vi "Check BOM against Inventory.vi"() -> ()   [LabVIEW 2013]
panel:
  out "Report":string
  in  "Check":bool
  in  "BOM":path
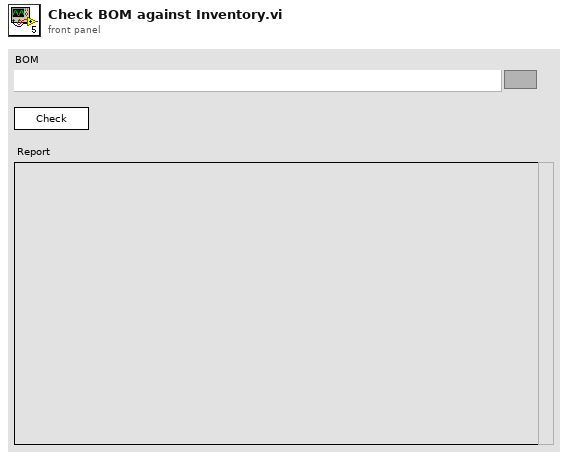
[diagram p1: front panel]
types:
  T1 = typedef "Display Component Line.ctl" = cluster{"Part Number":string, "Code (Value)":string, "Component Type":T2, "Component Subtype":T3, "Quantity":u32, "Add":T4, "Subtract":T5}
  T2 = typedef "Components.ctl" = enum16{"Resistor", "Capacitor", "Diode", "Voltage Regulator", "Transistors", "ICs", "Misc"}
  T3 = typedef "Component Sub Type.ctl" = enum16{"N/A", "Carbon", "Variable - Trimmer", "Variable - Pot", "Ceramic", "Electrolitic", "Zenner", "TO-92", "TO-220", "NPN", "PNP", "CMOS", "Processor"}
  T4 = typedef "Add Button.ctl" = bool
  T5 = typedef "Subtract Button.ctl" = bool
  T6 = typedef "BOM Item.ctl" = cluster{"Quantity":i32, "Component Type":string, "Component Value":string, "Component Type Estimate":T2, "Component Subtype Estimate":T3}
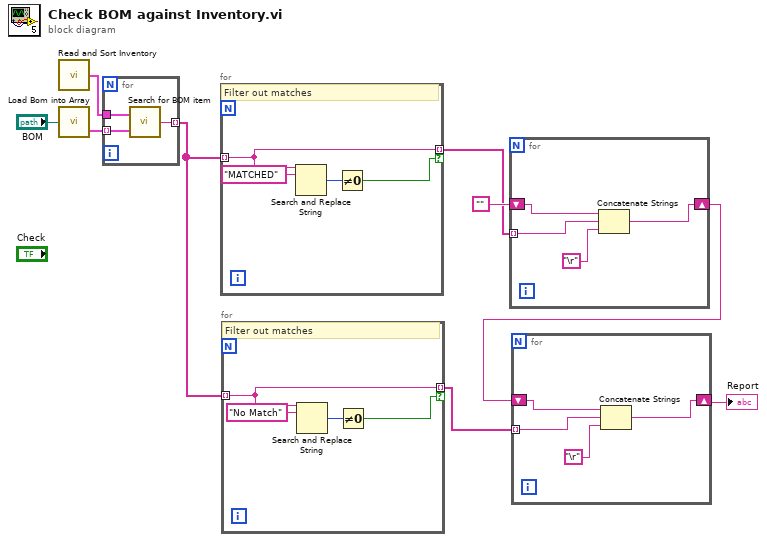
[diagram p0: block diagram]
diagram:
  n1 = call "Read and Sort Inventory.vi"() -> ("Array"=w7:T1[])  [unwired: 1 in]
  n2 = call "Load Bom into Array.vi"("BOM"="BOM") -> ("Cluster Bom"=w8:T6[])  [unwired: 1 out]
  n3 = for {
    tunnel: w8 -> [w12] mode=indexing
    tunnel: w7 -> [w11]
    tunnel: [w10] -> w6 mode=indexing
    n4 = call "Search for BOM item.vi"("BOM Item"=w12, "Inventory"=w11) -> ("Line Item Report"=w10:string)
  }
  n5 = for {
    tunnel: w6 -> [w14] mode=indexing
    tunnel: [w14] -> w4 mode=indexing if=w13
    # "Filter out matches"
    n6 = Search and Replace String(input string=w14, search string="MATCHED") -> (number of replacements=w15:i32)  [unwired: 6 in, 3 out]
    n7 = Not Equal To 0?(x=w15) -> (x != 0?=w13:bool)
  }
  n8 = for {
    tunnel: w6 -> [w18] mode=indexing
    tunnel: [w18] -> w3 mode=indexing if=w17
    # "Filter out matches"
    n9 = Search and Replace String(input string=w18, search string="No Match") -> (number of replacements=w19:i32)  [unwired: 6 in, 3 out]
    n10 = Not Equal To 0?(x=w19) -> (x != 0?=w17:bool)
  }
  n11 = for {
    shift-right: [w21] -> w2
    shift-left: "" -> [w24]
    tunnel: w4 -> [w23] mode=indexing
    n12 = Concatenate Strings(w24, w23, "\r") -> (w21:string)
  }
  n13 = for {
    shift-right: [w25] -> w1
    shift-left: w2 -> [w28]
    tunnel: w3 -> [w27] mode=indexing
    n14 = Concatenate Strings(w28, w27, "\r") -> (w25:string)
  }
  "Report" <- w1
